vi "BCU诊断标定.vi"(8 "CAN端口":u16(ring), 9 "设备索引号":u16(ring), 10 "CAN卡类型":u32(ring)=21, 11 "Myindex":dbl=1.0) -> (3 "成功":bool)   [LabVIEW 2013] (continued)
                              n3534 = control-ref of="项目信息"() -> (w5018:refnum<vi>)
                              n3535 = for {
                                N: w5011 -> [_]
                                tunnel: [""] -> w5017 mode=indexing
                              }
                              n3536 = Multiply(x=u8 2, y=w5012) -> (x*y=w5014:dbl)
                              n3537 = Add(x=w5014, y=u8 22) -> (x+y=w5010:dbl)
                              n3538 = call "表格数据输入-8.6.vi"("行数"=w5010, "列数"=u32 1, "字符串数组"=w5017, "表格引用"=w5018) -> ()  [unwired: 8 in]
                            }
                            frame "温度起始值" {
                              n3539 = local read "从板个数"() -> (w5022:dbl)
                              n3540 = Increment(x=w5022) -> (x+1=w5021:dbl)
                              n3541 = control-ref of="项目信息"() -> (w5028:refnum<vi>)
                              n3542 = for {
                                N: w5021 -> [_]
                                tunnel: [""] -> w5027 mode=indexing
                              }
                              n3543 = Multiply(x=u8 3, y=w5022) -> (x*y=w5024:dbl)
                              n3544 = Add(x=w5024, y=u8 23) -> (x+y=w5020:dbl)
                              n3545 = call "表格数据输入-8.6.vi"("行数"=w5020, "列数"=u32 1, "字符串数组"=w5027, "表格引用"=w5028) -> ()  [unwired: 8 in]
                            }
                            frame "保险位置" {
                              n3546 = local read "从板个数"() -> (w5032:dbl)
                              n3547 = control-ref of="项目信息"() -> (w5038:refnum<vi>)
                              n3548 = for {
                                N: 10 -> [_]
                                tunnel: [""] -> w5037 mode=indexing
                              }
                              n3549 = Multiply(x=u8 4, y=w5032) -> (x*y=w5034:dbl)
                              n3550 = Add(x=w5034, y=u8 24) -> (x+y=w5031:dbl)
                              n3551 = call "表格数据输入-8.6.vi"("行数"=w5031, "列数"=u32 1, "字符串数组"=w5037, "表格引用"=w5038) -> ()  [unwired: 8 in]
                            }
                            frame "电池额定实际容量" {
                              w5040 = 0.0 ("值")
                              n3552 = control-ref of="电池实际容量(A)"() -> (w5041:refnum<vi>)
                              n3553 = control-ref of="电池额定容量(A)"() -> (w5042:refnum<vi>)
                              n3554 = property class="DigNum (严格)"(reference=w5041, "Value"=w5040) -> ()  [unwired: 1 in, 2 out]
                              n3555 = property class="DigNum (严格)"(reference=w5042, "Value"=w5040) -> ()  [unwired: 1 in, 2 out]
                            }
                            frame "SOC" {
                              n3556 = control-ref of="SOC(%)"() -> (w5043:refnum<vi>)
                              n3557 = property class="DigNum (严格)"(reference=w5043, "Value"=0.0 ("值")) -> ()  [unwired: 1 in, 2 out]
                            }
                            frame "配置文件版本" {
                              n3558 = control-ref of="配置文件版本"() -> (w5045:refnum<vi>)
                              n3559 = property class="Str"(reference=w5045, "Value"="" ("值")) -> ()  [unwired: 1 in, 2 out]
                            }
                            frame "参数修改记录" {
                              n3560 = control-ref of="使用者"() -> (w5048:refnum<vi>)
                              n3561 = control-ref of="系统时钟"() -> (w5049:refnum<vi>)
                              n3562 = property class="DigNum (严格)"(reference=w5048, "Value"=0.0 ("值")) -> ()  [unwired: 1 in, 2 out]
                              n3563 = property class="Str"(reference=w5049, "Value"="" ("值")) -> ()  [unwired: 1 in, 2 out]
                            }
                            frame "校正时钟" {
                              n3564 = control-ref of="系统时钟"() -> (w5051:refnum<vi>)
                              n3565 = property class="Str"(reference=w5051, "Value"="" ("值")) -> ()  [unwired: 1 in, 2 out]
                            }
                            frame "车牌号" {
                              n3566 = control-ref of="车架(牌)号"() -> (w5053:refnum<vi>)
                              n3567 = property class="Str"(reference=w5053, "Value"="" ("值")) -> ()  [unwired: 1 in, 2 out]
                            }
                            frame "SOH" {
                              n3568 = control-ref of="SOH(%)"() -> (w5056:refnum<vi>)
                              n3569 = property class="DigNum (严格)"(reference=w5056, "Value"=0.0 ("值")) -> ()  [unwired: 1 in, 2 out]
                            }
                            frame "一级故障阀值" {
                              n3570 = local write "一级故障"(T10 {"总电压过高"=0.0, "整组电压不均衡"=0.0, "SOC过高"=0.0, "单体电压过高"=0.0, "总电压过低"=0.0, "温度过高"=0.0, "温度过低"=0.0, "单组电压不均衡"=0.0, "整组温度不均衡"=0.0, "单组温度不均衡"=0.0, "单体电压过低"=0.0, "充电电流过高"=0.0, "放电电流过高"=0.0, "SOC过低"=0.0, "内阻过大"=0.0, "极柱温度过高"=0.0, "SOH过低"=0.0} ("一级故障")) -> ()
                            }
                            frame "二级故障阀值" {
                              n3571 = local write "一级故障 2"(T10 {"总电压过高"=0.0, "整组电压不均衡"=0.0, "SOC过高"=0.0, "单体电压过高"=0.0, "总电压过低"=0.0, "温度过高"=0.0, "温度过低"=0.0, "单组电压不均衡"=0.0, "整组温度不均衡"=0.0, "单组温度不均衡"=0.0, "单体电压过低"=0.0, "充电电流过高"=0.0, "放电电流过高"=0.0, "SOC过低"=0.0, "内阻过大"=0.0, "极柱温度过高"=0.0, "SOH过低"=0.0} ("一级故障")) -> ()
                            }
                            frame "三级故障阀值" {
                              n3572 = local write "一级故障 3"(T10 {"总电压过高"=0.0, "整组电压不均衡"=0.0, "SOC过高"=0.0, "单体电压过高"=0.0, "总电压过低"=0.0, "温度过高"=0.0, "温度过低"=0.0, "单组电压不均衡"=0.0, "整组温度不均衡"=0.0, "单组温度不均衡"=0.0, "单体电压过低"=0.0, "充电电流过高"=0.0, "放电电流过高"=0.0, "SOC过低"=0.0, "内阻过大"=0.0, "极柱温度过高"=0.0, "SOH过低"=0.0} ("一级故障")) -> ()
                            }
                            frame "加热控制参数" {
                              n3573 = local write "加热控制参数"(T11 {"风机开启温度"=0.0, "风机关闭温度"=0.0, "加热开启温度"=0.0, "加热关闭温度"=0.0, "风机开启温差"=0.0, "风机关闭温差"=0.0, "加热关闭温差"=0.0} ("加热控制参数")) -> ()
                            }
                            frame "充电控制参数" {
                              n3574 = local write "一级故障 5"(T12 {"最大允许单体电压"=0.0, "最大允许总电压"=0.0, "最小允许单体电压"=0.0, "最大允许充电电流"=0.0, "最小允许充电电流"=0.0, "最大允许充电温度"=0.0, "最小允许充电温度"=0.0, "电流步长"=0.0} ("一级故障 5")) -> ()
                            }
                            frame "电池信息1" {
                              w5062 = ""
                              w5063 = 0.0 ("电池串联")
                              n3575 = local read "电池信息"() -> (w5065:T13)
                              n3576 = Bundle By Name(cluster=w5065, "电池串联"=w5063, "电池并联"=w5063, "电池包额定容量"=w5063, "电池包额定能量(kWh)"=w5063, "电池包额定总电压"=w5063, "实际容量"=w5063, "电池厂家"=w5062, "电池类型"=w5062, "电池生产日期"=w5062) -> (w5064:T13)
                              n3577 = local write "电池信息"(w5064) -> ()
                            }
                            frame "电池包组号" {
                              n3578 = local read "电池信息"() -> (w5068:T13)
                              n3579 = Bundle By Name(cluster=w5068, "电池包组号"="") -> (w5067:T13)
                              n3580 = local write "电池信息"(w5067) -> ()
                            }
                            frame "充放电安时" {
                              w5069 = 0.0 ("累计充电总安时")
                              n3581 = local read "电池信息"() -> (w5071:T13)
                              n3582 = Bundle By Name(cluster=w5071, "累计充电总安时"=w5069, "累计放电总安时"=w5069) -> (w5070:T13)
                              n3583 = local write "电池信息"(w5070) -> ()
                            }
                            frame "电池充放电次数" {
                              w5072 = 0.0 ("累计充电总安时")
                              n3584 = local read "电池信息"() -> (w5074:T13)
                              n3585 = Bundle By Name(cluster=w5074, "电池充满次数"=w5072, "电池放空次数"=w5072, "电池充电次数"=w5072) -> (w5073:T13)
                              n3586 = local write "电池信息"(w5073) -> ()
                            }
                          }
                        }
                        frame "从板" {
                          n3587 = case shown="\"加热控制参数\"" w5075 {
                            frame "假", Default {
                            }
                            frame "电压起始值" {
                              n3588 = control-ref of="项目信息 2"() -> (w5077:refnum<vi>)
                              n3589 = for {
                                N: 1 -> [_]
                                tunnel: [""] -> w5080 mode=indexing
                              }
                              n3590 = call "表格数据输入-8.6.vi"("行数"=u32 0, "列数"=u32 1, "字符串数组"=w5080, "表格引用"=w5077) -> ()  [unwired: 8 in]
                            }
                            frame "通道电压节数" {
                              n3591 = control-ref of="项目信息 2"() -> (w5082:refnum<vi>)
                              n3592 = for {
                                N: 5 -> [_]
                                tunnel: [""] -> w5086 mode=indexing
                              }
                              n3593 = call "表格数据输入-8.6.vi"("行数"=u32 22, "列数"=u32 1, "字符串数组"=w5086, "表格引用"=w5082) -> ()  [unwired: 8 in]
                            }
                            frame "保险位置" {
                              n3594 = control-ref of="项目信息 2"() -> (w5088:refnum<vi>)
                              n3595 = for {
                                N: 20 -> [_]
                                tunnel: [""] -> w5092 mode=indexing
                              }
                              n3596 = call "表格数据输入-8.6.vi"("行数"=u32 2, "列数"=u32 1, "字符串数组"=w5092, "表格引用"=w5088) -> ()  [unwired: 8 in]
                            }
                            frame "温度起始值" {
                              n3597 = control-ref of="项目信息 2"() -> (w5094:refnum<vi>)
                              n3598 = for {
                                N: 1 -> [_]
                                tunnel: [""] -> w5098 mode=indexing
                              }
                              n3599 = call "表格数据输入-8.6.vi"("行数"=u32 1, "列数"=u32 1, "字符串数组"=w5098, "表格引用"=w5094) -> ()  [unwired: 8 in]
                            }
                            frame "加热控制参数" {
                              n3600 = local write "加热控制参数"(T11 {"风机开启温度"=0.0, "风机关闭温度"=0.0, "加热开启温度"=0.0, "加热关闭温度"=0.0, "风机开启温差"=0.0, "风机关闭温差"=0.0, "加热关闭温差"=0.0} ("加热控制参数")) -> ()
                            }
                            frame "一级故障阀值" {
                              n3601 = local write "一级故障 6"(T15 {"电压过高"=0.0, "电压过低"=0.0, "温度过高"=0.0, "温度过低"=0.0, "电压不均衡(V)"=0.0, "温度不均衡"=0.0, "SOC过低"=0.0} ("一级故障 6")) -> ()
                            }
                            frame "二级故障阀值" {
                              n3602 = local write "一级故障 7"(T15 {"电压过高"=0.0, "电压过低"=0.0, "温度过高"=0.0, "温度过低"=0.0, "电压不均衡(V)"=0.0, "温度不均衡"=0.0, "SOC过低"=0.0} ("一级故障 7")) -> ()
                            }
                            frame "三级故障阀值" {
                              n3603 = local write "一级故障 8"(T15 {"电压过高"=0.0, "电压过低"=0.0, "温度过高"=0.0, "温度过低"=0.0, "电压不均衡(V)"=0.0, "温度不均衡"=0.0, "SOC过低"=0.0} ("一级故障 7")) -> ()
                            }
                            frame "均衡参数" {
                              n3604 = local write "均衡参数"(T17 {"充电结束电压(90%)"=0.0, "充电结束电压(91%)"=0.0, "充电结束电压(92%)"=0.0, "充电结束电压(93%)"=0.0, "充电结束电压(94%)"=0.0, "均衡计算-电压高阀值1级"=0.0, "均衡计算-电压高阀值2级"=0.0, "均衡计算-电压低阀值1级"=0.0, "均衡计算-电压低阀值2级"=0.0, "均衡计算-最低电压阀值"=0.0, "均衡停止-最低电压阀值"=0.0, "均衡计算-电压极差阀值"=0.0, "充电结束电压(95%)"=0.0, "充电结束电压(96%)"=0.0, "充电结束电压(97%)"=0.0, "充电结束电压(98%)"=0.0, "充电结束电压(99%)"=0.0, "充电结束电压(100%)"=0.0} ("均衡参数")) -> ()
                            }
                            frame "均衡阀值" {
                              w5105 = sgl 0.0 ("均衡计算-电压高阀值1级")
                              n3605 = local read "均衡参数"() -> (w5106:T17)
                              n3606 = Bundle By Name(cluster=w5106, "均衡计算-电压高阀值1级"=w5105, "均衡计算-电压高阀值2级"=w5105, "均衡计算-电压低阀值1级"=w5105, "均衡计算-电压低阀值2级"=w5105, "均衡计算-最低电压阀值"=w5105, "均衡停止-最低电压阀值"=w5105, "均衡计算-电压极差阀值"=w5105) -> (w5107:T17)
                              n3607 = local write "均衡参数"(w5107) -> ()
                            }
                            frame "充电结束电压" {
                              w5108 = sgl 0.0 ("均衡计算-电压高阀值1级")
                              n3608 = local read "均衡参数"() -> (w5109:T17)
                              n3609 = Bundle By Name(cluster=w5109, "充电结束电压(90%)"=w5108, "充电结束电压(91%)"=w5108, "充电结束电压(92%)"=w5108, "充电结束电压(93%)"=w5108, "充电结束电压(94%)"=w5108, "充电结束电压(95%)"=w5108, "充电结束电压(96%)"=w5108, "充电结束电压(97%)"=w5108, "充电结束电压(98%)"=w5108, "充电结束电压(99%)"=w5108, "充电结束电压(100%)"=w5108) -> (w5110:T17)
                              n3610 = local write "均衡参数"(w5110) -> ()
                            }
                          }
                        }
                      }
                    }
                    frame #1 {
                      w5111 = FALSE ("流控帧")
                      w5112 = TRUE ("流控帧 2")
                      n3611 = global write "EV05全局变量1.vi" "写入超时"(w5111) -> ()
                      n3612 = global write "EV05全局变量1.vi" "流控帧"(w5111) -> ()
                      n3613 = local write "写?"(w5111) -> ()
                      n3614 = call <vilib>:"Set Busy.vi"("disable click? (T)"=w5111) -> ()  [unwired: 3 in, 8 out]
                      n3615 = local write "消除"(w5112) -> ()
                      n3616 = local write "控制1"(w5112) -> ()
                      n3617 = global write "EV05全局变量1.vi" "流控帧 2"(w5112) -> ()
                    }
                    frame #2 {
                      n3618 = Wait Until Next ms Multiple(millisecond multiple=u32 150 ("毫秒倍数")) -> ()  [unwired: 1 out]
                    }
                    frame #3 {
                      n3619 = local read "设备索引号"() -> (w5119:u16)
                      n3620 = local read "CAN卡类型"() -> (w5120:u32)
                      n3621 = local read "CAN端口"() -> (w5118:u16)
                      n3622 = stacked-sequence {
                        tunnel: w5120 -> [_ w5128]
                        tunnel: w5119 -> [_ w5127]
                        tunnel: w5118 -> [_ w5126]
                        tunnel: w5117 -> [_ w5125]
                        tunnel: w5116 -> [_ w5124]
                        tunnel: w5115 -> [_ w5123]
                        tunnel: w5114 -> [_ w5122]
                        frame #0 {
                        }
                        frame #1 {
                          n3623 = call "多帧发送机制(EV05).vi"("can卡类型"=w5128, "设备索引号"=w5127, "CAN端口"=w5126, "命令"=w5124, "板号"=w5123, "命令序号"=w5125, "输入数据"=w5122) -> ("错误输出"=w5121:errorcluster)  [unwired: 2 in, 10 out]
                          n3624 = call <vilib>:"Clear Errors.vi"("error in (no error)"=w5121) -> ()  [unwired: 6 in, 1 out]
                        }
                      }
                      "命令序号" <- w5117
                    }
                    frame #4 {
                      n3625 = while {
                        tunnel: [w5133] -> w5130
                        tunnel: [w5132] -> w5129
                        i -> [w5136]
                        stop <- w5133 stop-if-true
                        n3626 = local read "强制终止读写标记"() -> (w5131:bool)
                        n3627 = global read "EV05全局变量1.vi" "写入超时"() -> (w5132:bool)
                        n3628 = Greater Or Equal?(x=w5136, y=30) -> (x >= y?=w5134:bool)
                        n3629 = Compound Arithmetic op=OR(w5131, w5132, w5134) -> (w5133:bool)
                        n3630 = Wait Until Next ms Multiple(millisecond multiple=u32 100 ("毫秒倍数")) -> ()  [unwired: 1 out]
                      }
                    }
                    frame #5 {
                      n3631 = call <vilib>:"Unset Busy.vi"() -> ()  [unwired: 11 in, 1 out]
                      n3632 = case shown="假" w5138 {
                        tunnel: w5139 -> [w5142 _]
                        frame False {
                          n3633 = control-ref of="结果"() -> (w5141:refnum<vi>)
                          n3634 = Concatenate Strings(w5142, "     读取失败" ("字符串")) -> (w5144:string)
                          n3635 = Build Array(w5144) -> (w5140:string[])
                          n3636 = call "表格编辑.vi"("新元素/子数组"=w5140, "活动单元格:单元格背景色"=u32 16740749, "MCListbox引用句柄"=w5141) -> ()  [unwired: 9 out]
                        }
                        frame True {
                        }
                      }
                    }
                    frame #6 {
                      n3637 = Increment(x=w5148) -> (x+1=w5147:i32)
                      n3638 = Equal?(x=w5149, y=w5147) -> (x = y?=w5146:bool)
                      n3639 = case shown="真" w5146 {
                        frame False {
                        }
                        frame True {
                          n3640 = control-ref of="结果"() -> (w5151:refnum<vi>)
                          n3641 = Concatenate Strings("读取完成" ("字符串")) -> (w5153:string)
                          n3642 = Build Array(w5153) -> (w5150:string[])
                          n3643 = call "表格编辑.vi"("新元素/子数组"=w5150, "活动单元格:单元格背景色"=u32 21937, "MCListbox引用句柄"=w5151) -> ()  [unwired: 9 out]
                        }
                      }
                    }
                  }
                }
              }
            }
          }
          n3644 = stacked-sequence {
            tunnel: w4803 -> [_]
            frame #0 {
              n3645 = call <vilib>:"Unset Busy.vi"() -> ()  [unwired: 11 in, 1 out]
              n3646 = local write "强制终止读写标记"(FALSE ("强制停止")) -> ()
            }
          }
        }
        frame "全部读取" {
          n3647 = stacked-sequence {
            seq-local: [w5159 _ _] -> [_ _ w5714]
            seq-local: [w5158 _ _] -> [_ _ w5713]
            tunnel: [_ w5350 _] -> w5156
            frame #0 {
              n3648 = local read "主从选择"() -> (w5159:enum32{"主板", "从板"})
              n3649 = local read "路径"() -> (w5160:path)
              n3650 = Empty String/Path?(string/path=w5160) -> (empty?=w5158:bool)
              n3651 = disable-structure shown="禁用" {
                disable-tunnel: w5160 -> [w5163 _]
                disable-tunnel: w5158 -> [w5162 _]
                disable-tunnel: w5159 -> [w5161 _]
                frame Disabled {
                  n3652 = case shown="假" w5162 {
                    tunnel: w5163 -> [w5167 _]
                    tunnel: w5161 -> [w5166 _]
                    frame False {
                      n3653 = control-ref of="结果"() -> (w5164:refnum<vi>)
                      n3654 = call-poly <vilib>:"Read From Spreadsheet File.vi"("file path (dialog if empty)"=w5167) -> ("all rows"=w5165:string[][])  [unwired: 3 in, 7 out]
                      n3655 = case shown="\"主板\", 默认" w5166 {
                        tunnel: w5165 -> [w5169 w5264]
                        tunnel: w5164 -> [w5168 w5263]
                        frame "主板", Default {
                          n3656 = stacked-sequence {
                            tunnel: w5169 -> [w5178 w5202 w5259]
                            tunnel: w5168 -> [w5175 _ w5230]
                            frame #0 {
                              n3657 = Index Array(array=w5178, index (col)=3 ("禁用的索引 (列)")) -> (element=w5192:string[])  [unwired: 1 in]
                              n3658 = Index Array(array=w5178, index (col)=1 ("禁用的索引 (列)")) -> (element=w5198:string[])  [unwired: 1 in]
                              n3659 = Delete From Array(array=w5192, length=4 ("长度"), index=0 ("索引")) -> (deleted portion=w5189:string[], array with subset deleted=w5183:string[])
                              n3660 = Delete From Array(array=w5198, length=1 ("长度"), index=0 ("索引")) -> (deleted portion=w5195:string[], array with subset deleted=w5172:string[])
                              n3661 = Build Array("正在读取主板配置文件...") -> (w5176:string[])
                              n3662 = Index Array(array=w5183) -> (element #1=w5182:string, element #2=w5181:string, element #3=w5180:string, element #4=w5179:string)  [unwired: 4 in]
                              n3663 = for {
                                tunnel: w5189 -> [w5201] mode=indexing
                                tunnel: [w5200] -> w5188 mode=indexing
                                n3664 = Fract/Exp String To Number(string=w5201) -> (number=w5200:dbl)  [unwired: 4 out]
                              }
                              n3665 = Index Array(array=w5195) -> (element=w5194:string)  [unwired: 1 in]
                              n3666 = global write "读配置文件全局.vi" "表格输入"(w5172) -> ()
                              n3667 = call "表格编辑.vi"("新元素/子数组"=w5176, "活动单元格:单元格背景色"=u32 6618880, "MCListbox引用句柄"=w5175) -> ()  [unwired: 9 out]
                              n3668 = Decimal String To Number(string=w5194) -> (number=w5173:i32)  [unwired: 1 in, 2 out]
                              n3669 = global read "读配置文件全局.vi" "项目信息"() -> (w5171:T27)
                              n3670 = Index Array(array=w5188) -> (element #1=w5187:dbl, element #2=w5186:dbl, element #3=w5185:dbl, element #4=w5184:dbl)  [unwired: 4 in]
                              n3671 = global write "读配置文件全局.vi" "从板个数"(w5173) -> ()
                              n3672 = Bundle(cluster=w5171, "电池额定容量"=w5187, "电池实际容量"=w5186, "车牌号"=w5182, "配置文件版本"=w5181, "SOH"=w5184, "SOC"=w5185, "产品编号"=w5180, "系统时钟"=w5179) -> (w5170:T27)  [unwired: 1 out]
                              n3673 = global write "读配置文件全局.vi" "项目信息"(w5170) -> ()
                            }
                            frame #1 {
                              n3674 = Index Array(array=w5202, index (col)=3 ("禁用的索引 (列)")) -> (element=w5220:string[])  [unwired: 1 in]
                              n3675 = Index Array(array=w5202, index (col)=5 ("禁用的索引 (列)")) -> (element=w5214:string[])  [unwired: 1 in]
                              n3676 = for {
                                tunnel: w5214 -> [w5227] mode=indexing
                                tunnel: [w5226] -> w5213 mode=indexing
                                n3677 = Fract/Exp String To Number(string=w5227) -> (number=w5226:dbl)  [unwired: 4 out]
                              }
                              n3678 = Delete From Array(array=w5220, length=17 ("长度"), index=8 ("索引")) -> (deleted portion=w5218:string[])  [unwired: 1 out]
                              n3679 = for {
                                tunnel: w5218 -> [w5229] mode=indexing
                                tunnel: [w5228] -> w5216 mode=indexing
                                n3680 = Fract/Exp String To Number(string=w5229) -> (number=w5228:dbl)  [unwired: 4 out]
                              }
                              n3681 = global write "读配置文件全局.vi" "二级故障"(w5213) -> ()
                              n3682 = global write "读配置文件全局.vi" "一级故障"(w5216) -> ()
                              n3683 = Index Array(array=w5202, index (col)=7 ("禁用的索引 (列)")) -> (element=w5211:string[])  [unwired: 1 in]
                              n3684 = Index Array(array=w5202, index (col)=9 ("禁用的索引 (列)")) -> (element=w5208:string[])  [unwired: 1 in]
                              n3685 = for {
                                tunnel: w5211 -> [w5225] mode=indexing
                                tunnel: [w5224] -> w5210 mode=indexing
                                n3686 = Fract/Exp String To Number(string=w5225) -> (number=w5224:dbl)  [unwired: 4 out]
                              }
                              n3687 = for {
                                tunnel: w5208 -> [w5223] mode=indexing
                                tunnel: [w5222] -> w5207 mode=indexing
                                n3688 = Fract/Exp String To Number(string=w5223) -> (number=w5222:dbl)  [unwired: 4 out]
                              }
                              n3689 = Delete From Array(array=w5207, length=6 ("长度"), index=0 ("索引")) -> (deleted portion=w5204:dbl[], array with subset deleted=w5203:dbl[])
                              n3690 = global write "读配置文件全局.vi" "三级故障"(w5210) -> ()
                              n3691 = global write "读配置文件全局.vi" "加热控制参数"(w5204) -> ()
                              n3692 = global write "读配置文件全局.vi" "充电控制参数"(w5203) -> ()
                            }
                            frame #2 {
                              n3693 = call <vilib>:"Unset Busy.vi"() -> ()  [unwired: 2 in, 10 out]
                              n3694 = Index Array(array=w5259, index (col)=11 ("禁用的索引 (列)")) -> (element=w5256:string[])  [unwired: 1 in]
                              n3695 = Delete From Array(array=w5256, length=6 ("长度"), index=0 ("索引")) -> (deleted portion=w5238:string[], array with subset deleted=w5237:string[])
                              n3696 = for {
                                tunnel: w5237 -> [w5262] mode=indexing
                                tunnel: [w5261] -> w5255 mode=indexing
                                n3697 = Fract/Exp String To Number(string=w5262) -> (number=w5261:dbl)  [unwired: 4 out]
                              }
                              n3698 = Index Array(array=w5238) -> (element #1=w5254:string, element #2=w5253:string, element #3=w5252:string, element #4=w5251:string, element #5=w5250:string, element #6=w5249:string)  [unwired: 6 in]
                              n3699 = Index Array(array=w5255) -> (element #1=w5248:dbl, element #2=w5247:dbl, element #3=w5246:dbl, element #4=w5245:dbl, element #5=w5244:dbl, element #6=w5243:dbl, element #7=w5242:dbl, element #8=w5241:dbl, element #9=w5240:dbl, element #10=w5239:dbl, element #11=w5234:dbl)  [unwired: 11 in]
                              n3700 = global read "读配置文件全局.vi" "电池信息"() -> (w5236:T28)
                              n3701 = Build Array("配置文件读取完成") -> (w5232:string[])
                              n3702 = Bundle(cluster=w5236, "电池串联"=w5248, "电池并联"=w5247, "累计放电总安时"=w5245, "电池包额定容量"=w5244, "电池包额定能量"=w5243, "电池包额定总电压"=w5242, "累计充电总安时"=w5246, "电池充满次数"=w5241, "电池放空次数"=w5240, "电池充电次数"=w5239, "电池生产日期"=w5254, "电池厂家"=w5253, "电池类型"=w5252, "电池包组号"=w5251, "电池包产权标识"=w5250, "电池应用车型"=w5249, "实际容量"=w5234) -> (w5235:T28)
                              n3703 = call "表格编辑.vi"("新元素/子数组"=w5232, "活动单元格:单元格背景色"=u32 6618880, "MCListbox引用句柄"=w5230) -> ()  [unwired: 9 out]
                              n3704 = global write "读配置文件全局.vi" "电池信息"(w5235) -> ()
                            }
                          }
                        }
                        frame "从板" {
                          n3705 = stacked-sequence {
                            tunnel: w5264 -> [w5272 w5300 w5344]
                            tunnel: w5263 -> [w5269 _ w5320]
                            frame #0 {
                              n3706 = Index Array(array=w5272, index (col)=1 ("禁用的索引 (列)")) -> (element=w5282:string[])  [unwired: 1 in]
                              n3707 = Index Array(array=w5272, index (col)=3 ("禁用的索引 (列)")) -> (element=w5276:string[])  [unwired: 1 in]
                              n3708 = Delete From Array(array=w5282, length=1 ("长度"), index=0 ("索引")) -> (deleted portion=w5279:string[], array with subset deleted=w5266:string[])
                              n3709 = Delete From Array(array=w5276, length=6 ("长度"), index=0 ("索引")) -> (deleted portion=w5273:string[])  [unwired: 1 out]
                              n3710 = for {
                                tunnel: w5273 -> [w5285] mode=indexing
                                tunnel: [w5284] -> w5265 mode=indexing
                                i -> [w5286]
                                n3711 = Fract/Exp String To Number(string=w5285, default (0 dbl)=w5286) -> (number=w5284:i32)  [unwired: 3 out]
                              }
                              n3712 = Index Array(array=w5279) -> (element=w5278:string)  [unwired: 1 in]
                              n3713 = global write "读配置文件全局2.vi" "表格"(w5266) -> ()
                              n3714 = Build Array("正在读取从板配置文件...") -> (w5270:string[])
                              n3715 = Decimal String To Number(string=w5278) -> (number=w5267:i32)  [unwired: 1 in, 2 out]
                              n3716 = call "表格编辑.vi"("新元素/子数组"=w5270, "活动单元格:单元格背景色"=u32 6618880, "MCListbox引用句柄"=w5269) -> ()  [unwired: 9 out]
                              n3717 = global write "读配置文件全局2.vi" "加热控制参数"(w5265) -> ()
                              n3718 = global write "读配置文件全局2.vi" "从板板号"(w5267) -> ()
                            }
                            frame #1 {
                              n3719 = Index Array(array=w5300, index (col)=3 ("禁用的索引 (列)")) -> (element=w5290:string[])  [unwired: 1 in]
                              n3720 = Array Subset(array=w5290, index=6 ("索引"), length=7 ("长度")) -> (w5297:string[])
                              n3721 = Array Subset(array=w5290, index=13 ("索引"), length=7 ("长度")) -> (w5296:string[])
                              n3722 = Array Subset(array=w5290, index=20 ("索引"), length=7 ("长度")) -> (w5291:string[])
                              n3723 = for {
                                tunnel: w5297 -> [w5307] mode=indexing
                                tunnel: [w5306] -> w5287 mode=indexing
                                n3724 = Fract/Exp String To Number(string=w5307) -> (number=w5306:dbl)  [unwired: 4 out]
                              }
                              n3725 = for {
                                tunnel: w5296 -> [w5305] mode=indexing
                                tunnel: [w5304] -> w5288 mode=indexing
                                n3726 = Fract/Exp String To Number(string=w5305) -> (number=w5304:dbl)  [unwired: 4 out]
                              }
                              n3727 = for {
                                tunnel: w5291 -> [w5303] mode=indexing
                                tunnel: [w5302] -> w5289 mode=indexing
                                n3728 = Fract/Exp String To Number(string=w5303) -> (number=w5302:dbl)  [unwired: 4 out]
                              }
                              n3729 = global write "读配置文件全局2.vi" "一级故障阀值"(w5287) -> ()
                              n3730 = global write "读配置文件全局2.vi" "二级故障阀值"(w5288) -> ()
                              n3731 = global write "读配置文件全局2.vi" "三级故障阀值"(w5289) -> ()
                            }
                            frame #2 {
                              n3732 = Index Array(array=w5344, index (col)=5 ("禁用的索引 (列)")) -> (element=w5342:string[])  [unwired: 1 in]
                              n3733 = Delete From Array(array=w5342, length=1 ("长度"), index=16 ("索引")) -> (deleted portion=w5338:string[], array with subset deleted=w5339:string[])
                              n3734 = for {
                                tunnel: w5339 -> [w5347] mode=indexing
                                tunnel: [w5346] -> w5343 mode=indexing
                                n3735 = Fract/Exp String To Number(string=w5347) -> (number=w5346:dbl)  [unwired: 4 out]
                              }
                              n3736 = Index Array(array=w5343) -> (element #1=w5337:dbl, element #2=w5336:dbl, element #3=w5335:dbl, element #4=w5334:dbl, element #5=w5333:dbl, element #6=w5332:dbl, element #7=w5331:dbl, element #8=w5330:dbl, element #9=w5329:dbl, element #10=w5328:dbl, element #11=w5327:dbl, element #12=w5318:dbl, element #13=w5326:dbl, element #14=w5325:dbl, element #15=w5324:dbl, element #16=w5323:dbl, element #17=w5316:dbl, element #18=w5315:dbl, element #19=w5314:dbl, element #20=w5313:dbl, element #21=w5312:dbl, element #22=w5311:dbl)  [unwired: 22 in]
                              n3737 = Build Array("配置文件读取完成") -> (w5321:string[])
                              n3738 = Index Array(array=w5338, index=22 ("索引")) -> (element=w5317:string)
                              n3739 = global read "读配置文件全局2.vi" "电池组信息"() -> (w5309:T29)
                              n3740 = call "表格编辑.vi"("新元素/子数组"=w5321, "活动单元格:单元格背景色"=u32 6618880, "MCListbox引用句柄"=w5320) -> ()  [unwired: 9 out]
                              n3741 = Bundle(cluster=w5309, "电池类型"=w5337, "电池厂家"=w5336, "电池地区"=w5335, "电池组序号"=w5334, "电池包串联数"=w5333, "电池包并联数"=w5332, "电池包安时数"=w5331, "电池包序号"=w5330, "充电次数"=w5329, "充满电时间"=w5328, "放空时间"=w5327, "车牌号"=w5317, "最大允许单体电压"=w5318, "最大允许总电压"=w5326, "最大允许温度"=w5325, "最小允许温度"=w5324, "最大允许充电电流"=w5323, "最小允许充电电流"=w5316, "最小允许单体电压"=w5315, "电流步长"=w5314, "SOC"=w5313, "充电总安时"=w5312, "放电总这时"=w5311) -> (w5308:T29)
                              n3742 = call <vilib>:"Unset Busy.vi"() -> ()  [unwired: 2 in, 10 out]
                              n3743 = global write "读配置文件全局2.vi" "电池组信息"(w5308) -> ()
                            }
                          }
                        }
                      }
                    }
                    frame True {
                    }
                  }
                }
                frame Enabled {
                }
              }
              n3744 = case shown="\"从板\"" w5159 {
                frame "主板", Default {
                  w5348 = FALSE
                  n3745 = global write "读配置文件全局.vi" "SOC判定"(w5348) -> ()
                  n3746 = global write "读配置文件全局.vi" "SOH判定"(w5348) -> ()
                  n3747 = global write "读配置文件全局.vi" "车牌号判定"(w5348) -> ()
                  n3748 = global write "读配置文件全局.vi" "电池信息1判定"(w5348) -> ()
                  n3749 = global write "读配置文件全局.vi" "保险位置判定"(w5348) -> ()
                  n3750 = global write "读配置文件全局.vi" "产品编号判定"(w5348) -> ()
                  n3751 = global write "读配置文件全局.vi" "充放电安时判定"(w5348) -> ()
                  n3752 = global write "读配置文件全局.vi" "从板个数判定"(w5348) -> ()
                  n3753 = global write "读配置文件全局.vi" "电池包组号判定"(w5348) -> ()
                  n3754 = global write "读配置文件全局.vi" "电压个数判定"(w5348) -> ()
                  n3755 = global write "读配置文件全局.vi" "电压起始值判定"(w5348) -> ()
                  n3756 = global write "读配置文件全局.vi" "二级故障判定"(w5348) -> ()
                  n3757 = global write "读配置文件全局.vi" "三级故障判定"(w5348) -> ()
                  n3758 = global write "读配置文件全局.vi" "通道电压数判定"(w5348) -> ()
                  n3759 = global write "读配置文件全局.vi" "温度个数判定"(w5348) -> ()
                  n3760 = global write "读配置文件全局.vi" "一级故障判定"(w5348) -> ()
                  n3761 = global write "读配置文件全局.vi" "温度起始值判定"(w5348) -> ()
                  n3762 = global write "读配置文件全局.vi" "充电控制参数判定"(w5348) -> ()
                  n3763 = global write "读配置文件全局.vi" "电池充放电次数判定"(w5348) -> ()
                  n3764 = global write "读配置文件全局.vi" "加热控制参数判定"(w5348) -> ()
                  n3765 = global write "读配置文件全局.vi" "配置文件版本判定"(w5348) -> ()
                  n3766 = global write "读配置文件全局.vi" "电池额定实际容量判定"(w5348) -> ()
                }
                frame "从板" {
                  w5349 = FALSE
                  n3767 = disable-structure shown="禁用" {
                    frame Disabled {
                      n3768 = global read "读配置文件全局2.vi" "充电次数时间判定"() -> ()  [unwired: 1 in]
                      n3769 = global read "读配置文件全局2.vi" "电池包信息1判定"() -> ()  [unwired: 1 in]
                      n3770 = global read "读配置文件全局2.vi" "电池包序号判定"() -> ()  [unwired: 1 in]
                      n3771 = global read "读配置文件全局2.vi" "充放电安时判定"() -> ()  [unwired: 1 in]
                      n3772 = global read "读配置文件全局2.vi" "车牌号判定"() -> ()  [unwired: 1 in]
                      n3773 = global read "读配置文件全局2.vi" "充电参数判定"() -> ()  [unwired: 1 in]
                      n3774 = global read "读配置文件全局2.vi" "保险位置判定"() -> ()  [unwired: 1 in]
                    }
                    frame Enabled {
                    }
                  }
                  n3775 = global write "读配置文件全局2.vi" "从板号判定"(w5349) -> ()
                  n3776 = global write "读配置文件全局2.vi" "通道电压判定"(w5349) -> ()
                  n3777 = global write "读配置文件全局2.vi" "保险位置判定"(w5349) -> ()
                  n3778 = global write "读配置文件全局2.vi" "二级故障判定"(w5349) -> ()
                  n3779 = global write "读配置文件全局2.vi" "三级故障判定"(w5349) -> ()
                  n3780 = global write "读配置文件全局2.vi" "一级故障判定"(w5349) -> ()
                  n3781 = global write "读配置文件全局2.vi" "电压起始值判定"(w5349) -> ()
                  n3782 = global write "读配置文件全局2.vi" "温度起始值判定"(w5349) -> ()
                }
              }
            }
            frame #1 {
              (unwired) "均衡参数"
              # "去掉加热控制信息 20140106"
              n3783 = local read "主从选择"() -> (w5353:enum32{"主板", "从板"})
              n3784 = case shown="\"主板\", 默认" w5353 {
                tunnel: [string[] ["项目信息", "一级故障阀值", "二级故障阀值", "三级故障阀值", "加热控制信息", "充电控制信息", "电池信息"] string[] ["从板信息", "一级故障阀值", "二级故障阀值", "三级故障阀值"]] -> w5352
                frame "主板", Default {
                }
                frame "从板" {
                }
              }
              n3785 = Array Size(array=w5352) -> (size(s)=w5351:i32)
              n3786 = for {
                tunnel: w5352 -> [w5369] mode=indexing
                tunnel: w5353 -> [w5357]
                tunnel: w5351 -> [w5361]
                tunnel: [w5356] -> w5350
                i -> [w5358]
                n3787 = case shown="\"主板\", 默认" w5357 {
                  tunnel: [w5665 w5693] -> w5363
                  tunnel: [w5664 w5694] -> w5364
                  tunnel: w5369 -> [w5661 w5690]
                  tunnel: [u8 0 ("板号") w5691] -> w5368
                  tunnel: [u8 0 ("板号") u8 0 ("板号")] -> w5367
                  tunnel: [w5660 w5689] -> w5365
                  frame "主板", Default {
                    n3788 = case shown="\"项目信息\"" w5661 {
                      tunnel: [_ u8[] [1, 2, 3, 4, 5, 6, 13, 8, 7, 9, 10, 11, 12] u8[] [1] u8[] [2] u8[] [3] u8[] [1] u8[] [2] u8[] [1, 2, 3] u8[] [1, 2, 3, 4]] -> w5665
                      tunnel: [_ u8 128 ("命令") u8 129 ("命令") u8 129 ("命令") u8 129 ("命令") u8 130 ("命令") u8 130 ("命令") u8 131 ("命令") u8 132 ("命令")] -> w5664
                      tunnel: [_ string[] ["产品编号", "电压个数", "通道电压数", "电压起始值", "温度个数", "温度起始值", "保险位置", "电池额定实际容量", "SOC", "配置文件版本", "参数修改记录", "车牌号", "SOH"] string[] ["一级故障阀值"] string[] ["二级故障阀值"] string[] ["三级故障阀值"] string[] ["加热控制参数"] string[] ["充电控制参数"] _ string[] ["电池信息1", "电池包组号", "充放电安时", "电池充放电次数"]] -> w5660
                      frame "假", Default {
                      }
                      frame "项目信息" {
                      }
                      frame "一级故障阀值" {
                      }
                      frame "二级故障阀值" {
                      }
                      frame "三级故障阀值" {
                      }
                      frame "加热控制信息" {
                      }
                      frame "充电控制信息" {
                      }
                      frame "历史信息" {
                      }
                      frame "电池信息" {
                      }
                    }
                  }
                  frame "从板" {
                    n3789 = case shown="\"从板信息\"" w5690 {
                      tunnel: [_ u8 0 ("命令") u8 2 ("命令") u8 2 ("命令") u8 2 ("命令") u8 3 ("命令") u8 6 ("命令")] -> w5694
                      tunnel: [_ u8[] [6, 1, 2, 3, 4, 5] u8[] [1] u8[] [2] u8[] [3] u8[] [1, 2, 3, 4, 5, 6, 7] u8[] [1, 2]] -> w5693
                      tunnel: [_ string[] ["从板号", "电压起始值", "通道电压节数", "保险位置", "温度起始值", "加热控制参数"] string[] ["一级故障阀值"] string[] ["二级故障阀值"] string[] ["三级故障阀值"] string[] ["电池包信息1", "电池包序号", "充放电安时", "充电次数时间", "SOC", "车牌号", "充电参数"] string[] ["均衡阀值", "充电结束电压"]] -> w5689
                      frame "假", Default {
                      }
                      frame "从板信息" {
                      }
                      frame "一级故障阀值" {
                      }
                      frame "二级故障阀值" {
                      }
                      frame "三级故障阀值" {
                      }
                      frame "快换参数" {
                      }
                      frame "均衡参数" {
                      }
                    }
                    n3790 = local read "从板号"() -> (w5691:u8)
                  }
                }
                n3791 = Increment(x=w5358) -> (x+1=w5360:i32)
                n3792 = Equal?(x=w5361, y=w5360) -> (x = y?=w5359:bool)
                n3793 = case shown="\"从板\"" w5357 {
                  tunnel: w5358 -> [w5631 w5645]
                  frame "主板", Default {
                    n3794 = case shown="0, 默认" w5631 {
                      tunnel: [T8."项目信息" ("主从板") T8."一级故障阀值" ("主从板") T8."二级故障阀值" ("主从板") T8."三级故障阀值" ("主从板") T8."控制参数" ("主从板") T8."电池信息" ("主从板")] -> w5630
                      frame 0, Default {
                        n3795 = local write "1"(TRUE ("1")) -> ()
                      }
                      frame 1 {
                        n3796 = local write "1 2"(TRUE ("1 2")) -> ()
                      }
                      frame 2 {
                        n3797 = local write "1 3"(TRUE ("1 3")) -> ()
                      }
                      frame 3 {
                        n3798 = local write "1 4"(TRUE ("1 4")) -> ()
                      }
                      frame 4, 5 {
                        n3799 = local write "1 5"(TRUE ("1 5")) -> ()
                      }
                      frame 6 {
                        n3800 = local write "1 11"(TRUE ("1 11")) -> ()
                      }
                    }
                    n3801 = local write "主板2"(w5630) -> ()
                  }
                  frame "从板" {
                    n3802 = case shown="4" w5645 {
                      tunnel: [T21."从板信息" ("等级 2") T21."从板信息" ("等级 2") T21."一级故障阀值" ("等级 2") T21."二级故障阀值" ("等级 2") T21."三级故障阀值" ("等级 2") T21."快换参数" ("等级 2") T14."均衡参数" ("等级 2")] -> w5644
                      frame 99, Default {
                        n3803 = local write "1 6"(TRUE ("1 6")) -> ()
                      }
                      frame 0 {
                        n3804 = local write "1 6"(TRUE ("1 6")) -> ()
                      }
                      frame 1 {
                        n3805 = local write "1 7"(TRUE ("1 7")) -> ()
                      }
                      frame 2 {
                        n3806 = local write "1 8"(TRUE ("1 8")) -> ()
                      }
                      frame 3 {
                        n3807 = local write "1 9"(TRUE ("1 9")) -> ()
                      }
                      frame 5 {
                        n3808 = local write "1 10"(TRUE ("1 10")) -> ()
                      }
                      frame 4 {
                        n3809 = local write "1 12"(TRUE ("1 10")) -> ()
                      }
                    }
                    n3810 = local write "等级 2"(w5644) -> ()
                  }
                }
                n3811 = Array Size(array=w5363) -> (size(s)=w5362:i32)
                n3812 = local write "命令"(w5364) -> ()
                n3813 = Build Array(w5367) -> (w5366:u8[])
                n3814 = while {
                  tunnel: w5364 -> [w5401]
                  tunnel: w5368 -> [w5400]
                  tunnel: w5366 -> [w5399]
                  tunnel: w5362 -> [w5395]
                  tunnel: w5359 -> [w5398]
                  tunnel: w5357 -> [w5392]
                  tunnel: [w5391] -> w5356
                  shift-right: [w5390] -> _
                  shift-left: w5365 -> [w5371]
                  shift-right: [w5381] -> _
                  shift-left: w5363 -> [w5370]
                  i -> [w5396]
                  stop <- w5391 stop-if-true
                  n3815 = local read "强制终止读写标记"() -> (w5387:bool)
                  n3816 = Array Size(array=w5371) -> (size(s)=w5389:i32)
                  n3817 = Increment(x=w5396) -> (x+1=w5397:i32)
                  n3818 = Greater Than 0?(x=w5389) -> (x > 0?=w5388:bool)
                  n3819 = Equal?(x=w5395, y=w5397) -> (x = y?=w5393:bool)
                  n3820 = Not(x=w5387) -> (.not. x?=w5386:bool)
                  n3821 = And(x=w5386, y=w5388) -> (x .and. y?=w5385:bool)
                  n3822 = Delete From Array(array=w5371, length=1 ("长度"), index=0 ("索引")) -> (deleted portion=w5377:string[], array with subset deleted=w5382:string[])
                  n3823 = Index Array(array=w5377, index=0 ("索引")) -> (element=w5375:string)
                  n3824 = Delete From Array(array=w5370, length=1 ("长度"), index=0 ("索引")) -> (deleted portion=w5373:u8[], array with subset deleted=w5378:u8[])
                  n3825 = Index Array(array=w5373, index=0 ("索引")) -> (element=w5372:u8)
                  n3826 = case shown="真" w5385 {
                    tunnel: w5401 -> [_ w5417]
                    tunnel: w5372 -> [_ w5416]
                    tunnel: w5400 -> [_ w5415]
                    tunnel: w5399 -> [_ w5414]
                    tunnel: w5375 -> [_ w5413]
                    tunnel: w5398 -> [_ w5412]
                    tunnel: w5393 -> [_ w5411]
                    tunnel: w5392 -> [_ w5410]
                    tunnel: [string[] [] w5406] -> w5390
                    tunnel: w5382 -> [_ w5409]
                    tunnel: [u8[] [] w5404] -> w5381
                    tunnel: w5378 -> [_ w5408]
                    tunnel: w5371 -> [_ w5407]
                    tunnel: w5370 -> [_ w5405]
                    frame False {
                    }
                    frame True {
                      n3827 = while {
                        tunnel: w5417 -> [w5433]
                        tunnel: w5416 -> [w5432]
                        tunnel: w5415 -> [w5431]
                        tunnel: w5414 -> [w5430]
                        tunnel: w5413 -> [w5428]
                        tunnel: w5412 -> [w5427]
                        tunnel: w5411 -> [w5426]
                        tunnel: w5410 -> [w5425]
                        tunnel: w5409 -> [w5421]
                        tunnel: w5408 -> [w5419]
                        tunnel: w5407 -> [w5422]
                        tunnel: [w5423] -> w5406
                        tunnel: w5405 -> [w5420]
                        tunnel: [w5418] -> w5404
                        i -> [w5424]
                        stop <- w5429 stop-if-true
                        n3828 = stacked-sequence {
                          seq-local: [_ _ _ _ w5580 _ _] -> [_ _ _ _ _ w5596 _]
                          tunnel: w5433 -> [_ _ _ w5572 _ _ _]
                          tunnel: w5432 -> [_ _ _ w5571 _ _ _]
                          tunnel: w5431 -> [_ _ _ w5570 _ _ _]
                          tunnel: w5430 -> [_ _ _ w5569 _ _ _]
                          tunnel: [_ _ _ _ w5581 _ _] -> w5429
                          tunnel: w5428 -> [w5435 _ _ _ _ w5595 _]
                          tunnel: w5427 -> [_ _ _ _ _ _ w5623]
                          tunnel: w5426 -> [_ _ _ _ _ _ w5621]
                          tunnel: w5425 -> [w5434 _ _ _ _ _ _]
                          tunnel: w5424 -> [_ _ _ _ _ _ _]
                          tunnel: [_ _ _ _ _ w5594 _] -> w5423
                          tunnel: w5422 -> [_ _ _ _ _ w5593 _]
                          tunnel: w5421 -> [_ _ _ _ _ w5592 _]
                          tunnel: w5420 -> [_ _ _ _ _ w5591 _]
                          tunnel: w5419 -> [_ _ _ _ _ w5590 _]
                          tunnel: [_ _ _ _ _ w5589 _] -> w5418
                          frame #0 {
                            n3829 = case shown="\"主板\", 默认" w5434 {
                              tunnel: w5435 -> [w5436 w5527]
                              frame "主板", Default {
                                n3830 = case shown="\"电池包组号\"" w5436 {
                                frame "假", Default {
                                }
                                frame "产品编号" {
                                n3831 = control-ref of="产品编号"() -> (w5438:refnum<vi>)
                                n3832 = property class="Str"(reference=w5438, "Value"="") -> ()  [unwired: 1 in, 2 out]
                                }
                                frame "电压个数" {
                                n3833 = local read "从板个数"() -> (w5439:dbl)
                                n3834 = control-ref of="项目信息"() -> (w5443:refnum<vi>)
                                n3835 = for {
                                N: w5439 -> [_]
                                tunnel: [""] -> w5442 mode=indexing
                                }
                                n3836 = call "表格数据输入-8.6.vi"("行数"=u32 0, "列数"=u32 1, "字符串数组"=w5442, "表格引用"=w5443) -> ()  [unwired: 8 in]
                                }
                                frame "通道电压数" {
                                n3837 = disable-structure shown="禁用" {
                                frame Disabled {
                                n3838 = control-ref of="项目信息"() -> (w5449:refnum<vi>)
                                n3839 = for {
                                N: 20 -> [_]
                                tunnel: [""] -> w5448 mode=indexing
                                }
                                n3840 = local read "从板个数"() -> (w5450:dbl)
                                n3841 = Increment(x=w5450) -> (x+1=w5446:dbl)
                                n3842 = call "表格数据输入-8.6.vi"("行数"=w5446, "列数"=u32 1, "字符串数组"=w5448, "表格引用"=w5449) -> ()  [unwired: 8 in]
                                }
                                frame Enabled {
                                }
                                }
                                }
                                frame "电压起始值" {
                                n3843 = disable-structure shown="禁用" {
                                frame Disabled {
                                n3844 = local read "从板个数"() -> (w5454:dbl)
                                n3845 = Increment(x=w5454) -> (x+1=w5453:dbl)
                                n3846 = control-ref of="项目信息"() -> (w5460:refnum<vi>)
                                n3847 = for {
                                N: w5453 -> [_]
                                tunnel: [""] -> w5459 mode=indexing
                                }
                                n3848 = Multiply(x=u8 1, y=w5454) -> (x*y=w5456:dbl)
                                n3849 = Add(x=w5456, y=u8 21) -> (x+y=w5452:dbl)
                                n3850 = call "表格数据输入-8.6.vi"("行数"=w5452, "列数"=u32 1, "字符串数组"=w5459, "表格引用"=w5460) -> ()  [unwired: 8 in]
                                }
                                frame Enabled {
                                }
                                }
                                }
                                frame "温度个数" {
                                n3851 = local read "从板个数"() -> (w5464:dbl)
                                n3852 = Increment(x=w5464) -> (x+1=w5463:dbl)
                                n3853 = control-ref of="项目信息"() -> (w5470:refnum<vi>)
                                n3854 = for {
                                N: w5463 -> [_]
                                tunnel: [""] -> w5469 mode=indexing
                                }
                                n3855 = Multiply(x=u8 2, y=w5464) -> (x*y=w5466:dbl)
                                n3856 = Add(x=w5466, y=u8 22) -> (x+y=w5462:dbl)
                                n3857 = call "表格数据输入-8.6.vi"("行数"=w5462, "列数"=u32 1, "字符串数组"=w5469, "表格引用"=w5470) -> ()  [unwired: 8 in]
                                }
                                frame "温度起始值" {
                                n3858 = disable-structure shown="禁用" {
                                frame Disabled {
                                n3859 = local read "从板个数"() -> (w5474:dbl)
                                n3860 = Increment(x=w5474) -> (x+1=w5473:dbl)
                                n3861 = control-ref of="项目信息"() -> (w5480:refnum<vi>)
                                n3862 = for {
                                N: w5473 -> [_]
                                tunnel: [""] -> w5479 mode=indexing
                                }
                                n3863 = Multiply(x=u8 3, y=w5474) -> (x*y=w5476:dbl)
                                n3864 = Add(x=w5476, y=u8 23) -> (x+y=w5472:dbl)
                                n3865 = call "表格数据输入-8.6.vi"("行数"=w5472, "列数"=u32 1, "字符串数组"=w5479, "表格引用"=w5480) -> ()  [unwired: 8 in]
                                }
                                frame Enabled {
                                }
                                }
                                }
                                frame "保险位置" {
                                n3866 = local read "从板个数"() -> (w5484:dbl)
                                n3867 = control-ref of="项目信息"() -> (w5490:refnum<vi>)
                                n3868 = for {
                                N: 10 -> [_]
                                tunnel: [""] -> w5489 mode=indexing
                                }
                                n3869 = Multiply(x=u8 4, y=w5484) -> (x*y=w5486:dbl)
                                n3870 = Add(x=w5486, y=u8 24) -> (x+y=w5483:dbl)
                                n3871 = call "表格数据输入-8.6.vi"("行数"=w5483, "列数"=u32 1, "字符串数组"=w5489, "表格引用"=w5490) -> ()  [unwired: 8 in]
                                }
                                frame "电池额定实际容量" {
                                w5492 = 0.0 ("值")
                                n3872 = control-ref of="电池实际容量(A)"() -> (w5493:refnum<vi>)
                                n3873 = control-ref of="电池额定容量(A)"() -> (w5494:refnum<vi>)
                                n3874 = property class="DigNum (严格)"(reference=w5493, "Value"=w5492) -> ()  [unwired: 1 in, 2 out]
                                n3875 = property class="DigNum (严格)"(reference=w5494, "Value"=w5492) -> ()  [unwired: 1 in, 2 out]
                                }
                                frame "SOC" {
                                n3876 = control-ref of="SOC(%)"() -> (w5495:refnum<vi>)
                                n3877 = property class="DigNum (严格)"(reference=w5495, "Value"=0.0 ("值")) -> ()  [unwired: 1 in, 2 out]
                                }
                                frame "配置文件版本" {
                                n3878 = control-ref of="配置文件版本"() -> (w5497:refnum<vi>)
                                n3879 = property class="Str"(reference=w5497, "Value"="" ("值")) -> ()  [unwired: 1 in, 2 out]
                                }
                                frame "参数修改记录" {
                                n3880 = control-ref of="使用者"() -> (w5500:refnum<vi>)
                                n3881 = control-ref of="系统时钟"() -> (w5501:refnum<vi>)
                                n3882 = property class="DigNum (严格)"(reference=w5500, "Value"=0.0 ("值")) -> ()  [unwired: 1 in, 2 out]
                                n3883 = property class="Str"(reference=w5501, "Value"="" ("值")) -> ()  [unwired: 1 in, 2 out]
                                }
                                frame "校正时钟" {
                                n3884 = control-ref of="系统时钟"() -> (w5503:refnum<vi>)
                                n3885 = property class="Str"(reference=w5503, "Value"="" ("值")) -> ()  [unwired: 1 in, 2 out]
                                }
                                frame "车牌号" {
                                n3886 = control-ref of="车架(牌)号"() -> (w5505:refnum<vi>)
                                n3887 = property class="Str"(reference=w5505, "Value"="" ("值")) -> ()  [unwired: 1 in, 2 out]
                                }
